vi "single callbyref.vi"() -> ()   [LabVIEW 2013]
uses:
  result/result.lvclass
  dispatcher/pool sizes.ctl
  result/result.lvclass/result.ctl
  result/get data.vi
  result/get error.vi
  result/get owning task.vi
  result/get subresults.vi
  dispatcher/thread pool.lvclass
  standard reporters/event reporter/event reporter.lvclass
  standard action/call by reference action/call function by reference.lvclass
panel:
  out "subresults":refnum<class "result.lvclass">[](array[class])
  out "owning task":string
  out "error":errorcluster
  out "data":variant
  out "Time":u32
  out "result":refnum<class "result.lvclass">
  out "error out":errorcluster
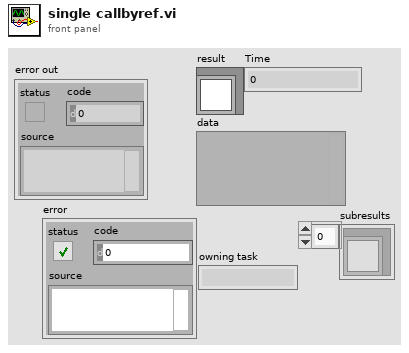
[diagram p1: front panel]
types:
  T1 = typedef "thread pool.lvclass/pool sizes.ctl" = cluster{"UI thread":u8, "standard":u8, "instrument I/O":u8, "data acquisition":u8, "other 1":u8, "other 2":u8}
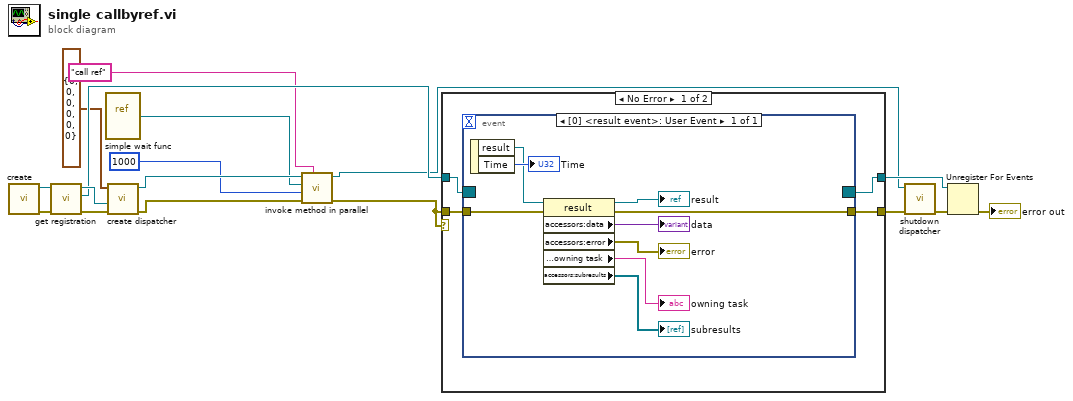
[diagram p0: block diagram]
diagram:
  n1 = call "create.vi"() -> ("error out"=w16:errorcluster, "event reporter out"=w17:refnum<class "event reporter.lvclass">)  [unwired: 10 in]
  n2 = call "get registration.vi"("error in"=w16, "event reporter in"=w17) -> ("error out"=w14:errorcluster, "result registration"=w13:refnum<event-registration>, "event reporter out"=w15:refnum<class "event reporter.lvclass">)  [unwired: 7 in]
  n3 = vi-ref "simple wait func.vi"() -> (w1:refnum<vi>)
  n4 = call "create dispatcher.vi"("error in"=w14, "default reporter"=w15, "initial pool sizes"=T1 {"UI thread"=0, "standard"=0, "instrument I/O"=0, "data acquisition"=0, "other 1"=0, "other 2"=0}) -> ("error out"=w5:errorcluster, "dispatcher"=w4:refnum<data-value>)  [unwired: 7 in]
  n5 = call "invoke method in parallel.vi"("ID"="call ref" ("action name"), "error in"=w5, "parameters"=1000, "VI in"=w1, "reporter"=w4) -> ("error out"=w7:errorcluster, "dispatcher out"=w11:refnum<data-value>)  [unwired: 5 in]
  n6 = case shown="No Error" w7 {
    tunnel: w13 -> [w21 w32]
    tunnel: [w20 w32] -> w12
    tunnel: [w19 w31] -> w8
    tunnel: w7 -> [w18 w31]
    frame No Error {
      n7 = event shown="[0] <result event>: User Event" {
        selector: w21 -> [_]
        dyn-events: [_] -> w20
        timeout: _ -> [_]
        tunnel: [w28] -> w19
        tunnel: w18 -> [w29]
        event User Event {
          n8 = event-data() -> ("result"=w27:refnum<class "result.lvclass">, "Time"=→"Time":u32)  [unwired: 1 in]
          n9 = property class="result"(reference=w27, error in=w29) -> (reference out=→"result":refnum<class "result.lvclass">, error out=w28:errorcluster, "accessors:data"=→"data":variant, "accessors:error"=→"error":errorcluster, "accessors:owning task"=→"owning task":string, "accessors:subresults"=→"subresults":refnum<class "result.lvclass">[])
        }
      }
    }
    frame Error {
    }
  }
  n10 = call "shutdown dispatcher.vi"("error in"=w8, "dispatcher"=w11) -> ("error out"=w10:errorcluster)  [unwired: 9 in]
  n11 = Unregister For Events(event registration refnum=w12, error in=w10) -> (error out=→"error out":errorcluster)
